vi "Untitled 2.vi"() -> ()   [LabVIEW 2020]
panel:
  out "standard error":string
  out "return code":i32
  out "error out":errorcluster
  out "standard output":string
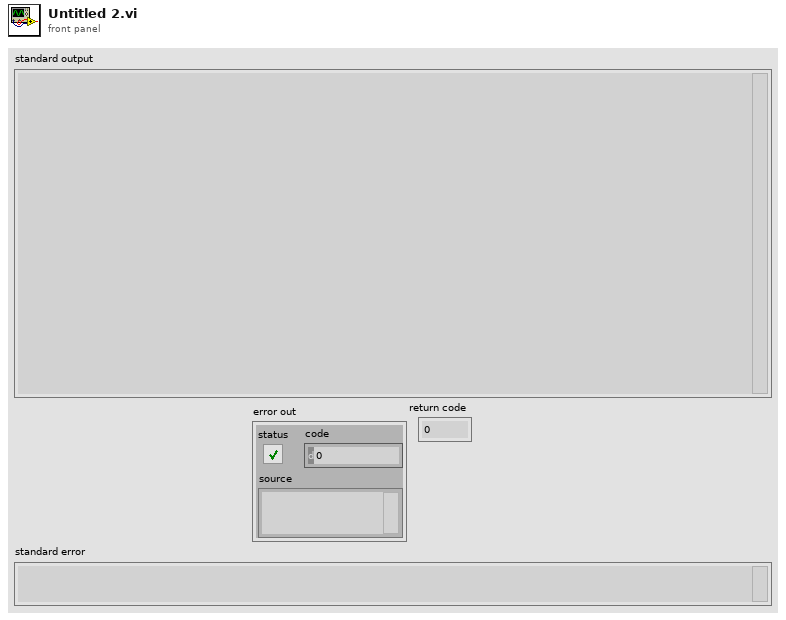
[diagram p1: front panel]
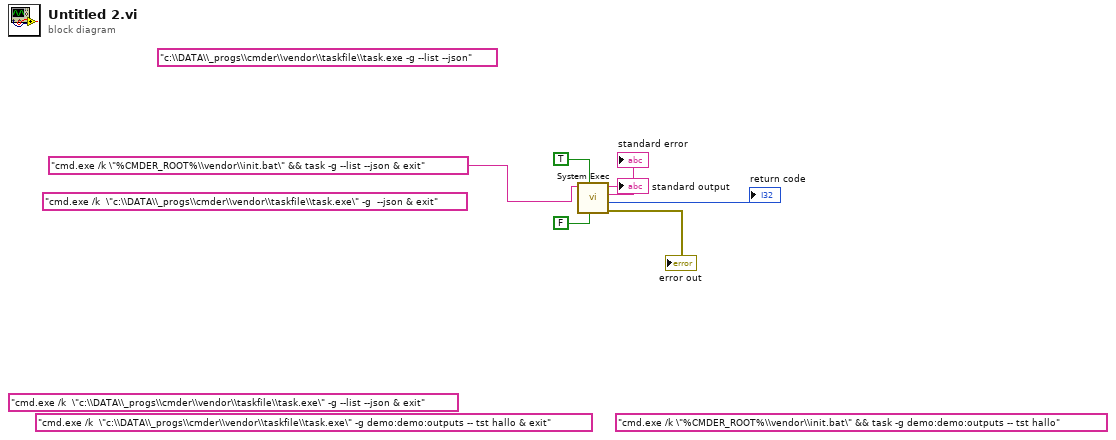
[diagram p0: block diagram]
diagram:
  (unwired) "cmd.exe /k  \"c:\\DATA\\_progs\\cmder\\vendor\\taskfile\\task.exe\" -g --list --json & exit" ("command line")
  (unwired) "cmd.exe /k  \"c:\\DATA\\_progs\\cmder\\vendor\\taskfile\\task.exe\" -g  --json & exit" ("command line")
  (unwired) "c:\\DATA\\_progs\\cmder\\vendor\\taskfile\\task.exe -g --list --json" ("command line")
  (unwired) "cmd.exe /k  \"c:\\DATA\\_progs\\cmder\\vendor\\taskfile\\task.exe\" -g demo:demo:outputs -- tst hallo & exit" ("command line")
  (unwired) "cmd.exe /k \"%CMDER_ROOT%\\vendor\\init.bat\" && task -g demo:demo:outputs -- tst hallo" ("command line")
  n1 = call <vilib>:"System Exec.vi"("run minimized? (F)"=FALSE, "wait until completion? (T)"=TRUE, "command line"="cmd.exe /k \"%CMDER_ROOT%\\vendor\\init.bat\" && task -g --list --json & exit") -> ("error out"=→"error out":errorcluster, "return code"=→"return code":i32, "standard error"=→"standard error":string, "standard output"=→"standard output":string)  [unwired: 5 in]
